vi "To BananaLeaf.vi"(10 "Properties":refnum<class "Properties.lvclass">) -> (3 "Leaf.Properties":refnum<class "Leaf.Properties.lvclass">)   [LabVIEW 2021, in "Banana.Caraya.lvlib" / "Leaf.Properties.lvclass"]
uses:
  Leaf.Properties.lvclass
  <vilib>/addons/_JKI Toolkits/Caraya/classes/Properties/Properties.lvclass
  Leaf.Properties.lvclass/Leaf.Properties.ctl
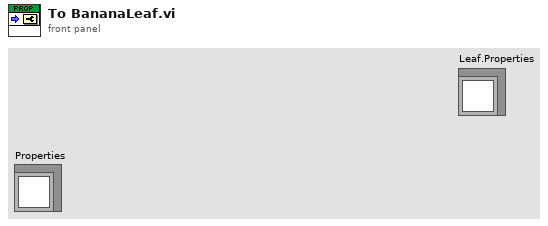
[diagram p1: front panel]
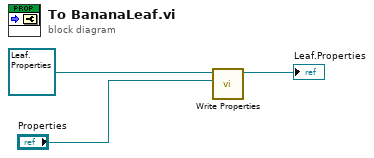
[diagram p0: block diagram]
diagram:
  n1 = call "Write Properties.vi"("Properties"="Properties", "Leaf.Properties in"=refnum<class "Leaf.Properties.lvclass"> refnum ("Leaf.Properties.Assert in")) -> ("Leaf.Properties out"=→"Leaf.Properties":refnum<class "Leaf.Properties.lvclass">)  [unwired: 9 in]
